vi "Hand Type.vi"(8 "error in (no error)":errorcluster, 11 "Hand In":refnum<class "Hand.lvclass">) -> (0 "error out":errorcluster, 2 "Score":T1(ring), 3 "Hand Out":refnum<class "Hand.lvclass">)   [LabVIEW 2020, in "Hand.lvclass"]
uses:
  Hand.lvclass
  Hand.lvclass/Hand.ctl
  a02ecccc-9047-47c4-92f0-a35d10906413.vi
  3f593b3f-7ea3-4136-9a25-4e23da202726.vi
  <vilib>/Comparison/Equal/Equal Functor/Equal Functor.lvclass
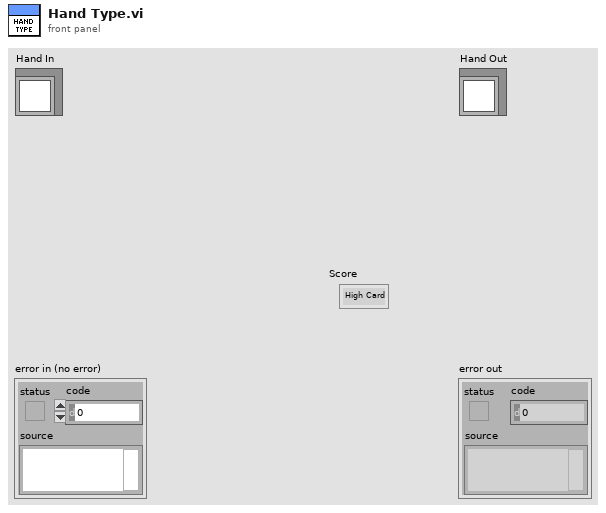
[diagram p1: front panel]
types:
  T1 = enum16{"High Card", "One Pair", "Two Pairs", "Three of a Kind", "Full House", "Four of a Kind", "Five of a Kind"}
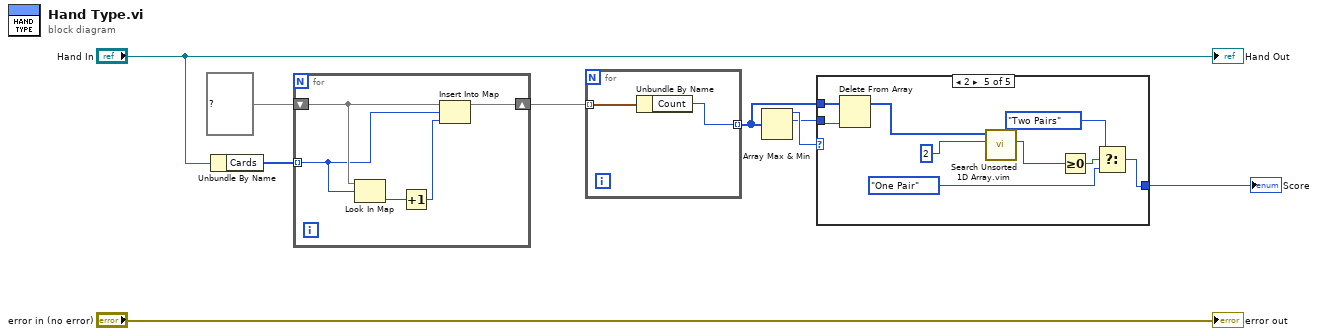
[diagram p0: block diagram]
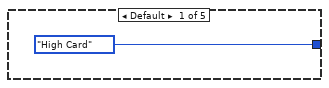
[diagram p2: hidden frame]
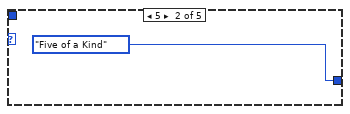
[diagram p3: hidden frame]
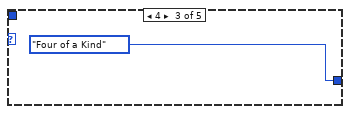
[diagram p4: hidden frame]
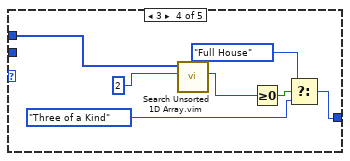
[diagram p5: hidden frame]
diagram:
  n1 = Unbundle By Name("Hand In") -> ("Cards"=w6:u8[])
  n2 = for {
    shift-right: [w10] -> w5
    shift-left: map{u8, u8} {} ("map") -> [w14]
    tunnel: w6 -> [w13] mode=indexing
    n3 = Look In Map(map=w14, key=w13) -> (value=w12:u8)  [unwired: 1 in, 1 out]
    n4 = Increment(x=w12) -> (x+1=w11:u8)
    n5 = Insert Into Map(map in=w14, key=w13, value=w11) -> (map out=w10:map{u8, u8})  [unwired: 2 out]
  }
  n6 = for {
    tunnel: w5 -> [w16] mode=indexing
    tunnel: [w15] -> w2 mode=indexing
    n7 = Unbundle By Name(w16) -> ("Count"=w15:u8)
  }
  n8 = Array Max & Min(array=w2) -> (max value=w4:u8, max index (indices)=w1:i32)  [unwired: 2 out]
  n9 = case shown="2" w4 {
    tunnel: [T1."High Card" ("Score") T1."Five of a Kind" ("Score") T1."Four of a Kind" ("Score") w21 w30] -> w3
    tunnel: w2 -> [_ _ _ w26 w35]
    tunnel: w1 -> [_ _ _ _ w27]
    frame Default {
    }
    frame 5 {
    }
    frame 4 {
    }
    frame 3 {
      n10 = call "Search Unsorted 1D Array.vim"("element"=2 ("Count"), "unsorted 1D array"=w26) -> ("index of element"=w24:i32)  [unwired: 9 in]
      n11 = Greater Or Equal To 0?(x=w24) -> (x >= 0?=w23:bool)
      n12 = Select(t=T1."Full House", s=w23, f=T1."Three of a Kind" ("Score")) -> (s? t:f=w21:T1)
    }
    frame 2 {
      n13 = Delete From Array(array=w35, index=w27) -> (array with subset deleted=w28:u8[])  [unwired: 1 in, 1 out]
      n14 = call "Search Unsorted 1D Array.vim"("element"=2 ("Count"), "unsorted 1D array"=w28) -> ("index of element"=w33:i32)  [unwired: 9 in]
      n15 = Greater Or Equal To 0?(x=w33) -> (x >= 0?=w32:bool)
      n16 = Select(t=T1."Two Pairs", s=w32, f=T1."One Pair" ("Score")) -> (s? t:f=w30:T1)
    }
  }
  "Score" <- w3
  "error out" <- "error in (no error)"
  "Hand Out" <- "Hand In"
